vi "Set Tickbox Caption - Not Owned.vi"(8 "Error In":errorcluster, 11 "Tickbox Ref":refnum<vi>) -> (0 "Error Out":errorcluster)   [LabVIEW 2022 SP3]
doc: "<add documentation here>"
panel:
  # "Development\nControls or indicators that are useful for development or testing, but which are not outputs of the VI."
  # "Input\nInputs to the VI"
  # "Output\nOutputs of the VI"
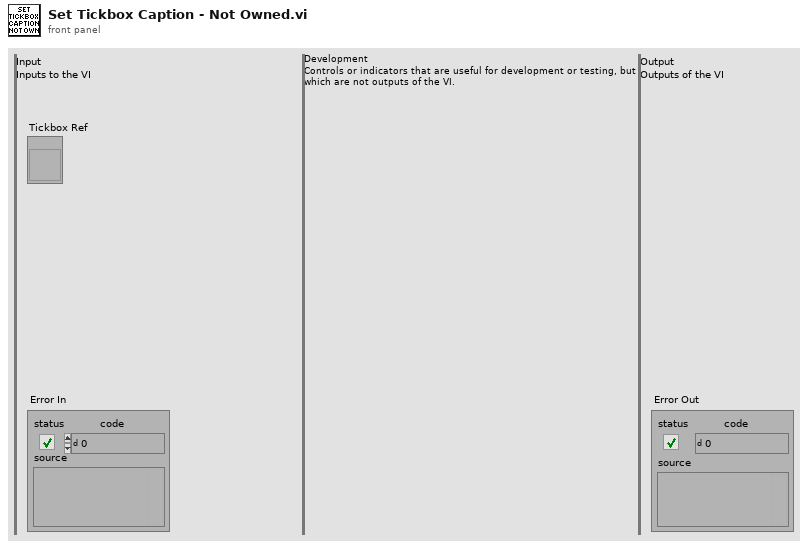
[diagram p1: front panel]
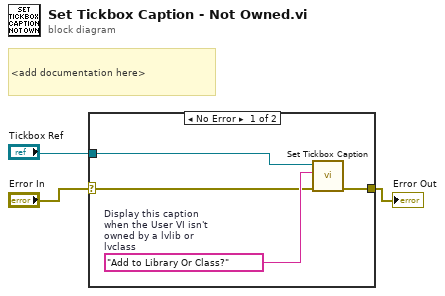
[diagram p0: block diagram]
diagram:
  # "<add documentation here>"
  n1 = case shown="No Error" "Error In" {
    selector: "Error In" -> [w6 w8]
    tunnel: [w5 w8] -> w2
    tunnel: "Tickbox Ref" -> [w4 _]
    frame No Error {
      w7 = "Add to Library Or Class?"  # Display this caption when the User VI isn't owned by a lvlib or lvclass
      n2 = call "Set Tickbox Caption.vi"("Error In"=w6, "Caption"=w7, "Tickbox Ref"=w4) -> ("Error Out"=w5:errorcluster)  [unwired: 8 in]
    }
    frame Error {
    }
  }
  "Error Out" <- w2
